vi "extra_waitlines_write.vi"(11 "address extra waitlines IN":u32) -> (0 "FIFO scan time out":bool, 2 "data":u32, 3 "address extra waitlines OUT":u32)   [LabVIEW 2010]
uses:
  <vilib>/rvi/DataTransferAndStorage/Container/XNode/niFpgaContainer.xnode
  <vilib>/rvi/DataTransferAndStorage/Container/Common/niFpgaContainerMethod.ctl
  <vilib>/rvi/DataTransferAndStorage/Container/Common/niFpgaTransferTypeControl.ctl
  <vilib>/rvi/interface/RandomDataEmulation/nirviRandomDataFPGAFIFO.vi
  <vilib>/rvi/interface/RandomDataEmulation/niFpgaRandomDataHandleErrors.vi
  <vilib>/rvi/Memory/Memory_Emulation/nirvimemoryEmulationManagerCache_GetValue.vi
  <vilib>/rvi/DataTransferAndStorage/Container/Common/niFpgaContainerGetUniqueNameForEmu.vi
  <vilib>/rvi/Memory/Memory_Emulation/nirvimemoryEmulationManagerCache_InsertValue.vi
  <vilib>/Utility/error.llb/Clear Errors.vi
  <vilib>/rvi/Memory/Memory_Emulation/nirvimemoryEmulationManagerCache_SetValue.vi
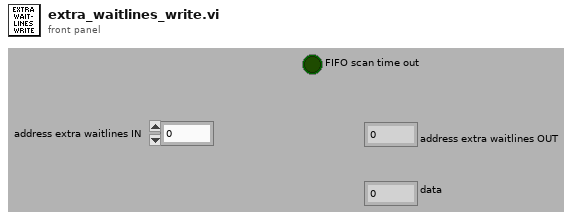
[diagram p1: front panel]
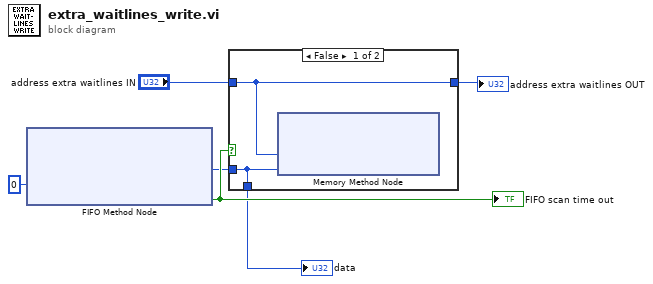
[diagram p0: block diagram]
diagram:
  n1 = xnode ("FIFO Method Node")("Timeout"=0) -> ("Element"=w2:u32, "Timed Out?"=w3:bool)  [unwired: 1 in, 1 out]
  "FIFO scan time out" <- w3
  n2 = case shown="False" w3 {
    tunnel: "address extra waitlines IN" -> [w8 w134]
    tunnel: [w8 w134] -> w5
    tunnel: w2 -> [w7 _]
    tunnel: [w7 _] -> w1
    frame False {
      n3 = xnode ("Memory Method Node")("Address"=w8, "Data"=w7) -> ()  [unwired: 1 in, 1 out]
    }
    frame True {
    }
  }
  "address extra waitlines OUT" <- w5
  "data" <- w1
